vi "DataStream_PC_Main Graph.vi"() -> ()   [LabVIEW 2020]
uses:
  4f3d7b8b-e590-4c89-bcad-6071a54aa44d.vi
  TypeDefs/Cluster_DataStream PC Map Data Set.ctl
panel:
  out "New Update":bool
  out "Cursor Y Diff":dbl
  out "Cursor Time Diff":dbl
  in  "Reset Data":bool
  in  "Pause":bool
  in  "Point Size":i32=2000
  in  "milliseconds to wait":u32=100
  out "Is Connected":bool
  out "Error":errorcluster
  out "error out":errorcluster
  out "XY Graph":cluster{dbl[], dbl[]}[](graph)
  in  "Stop":bool
  in  "Target IP Address":string="172.22.11.2"
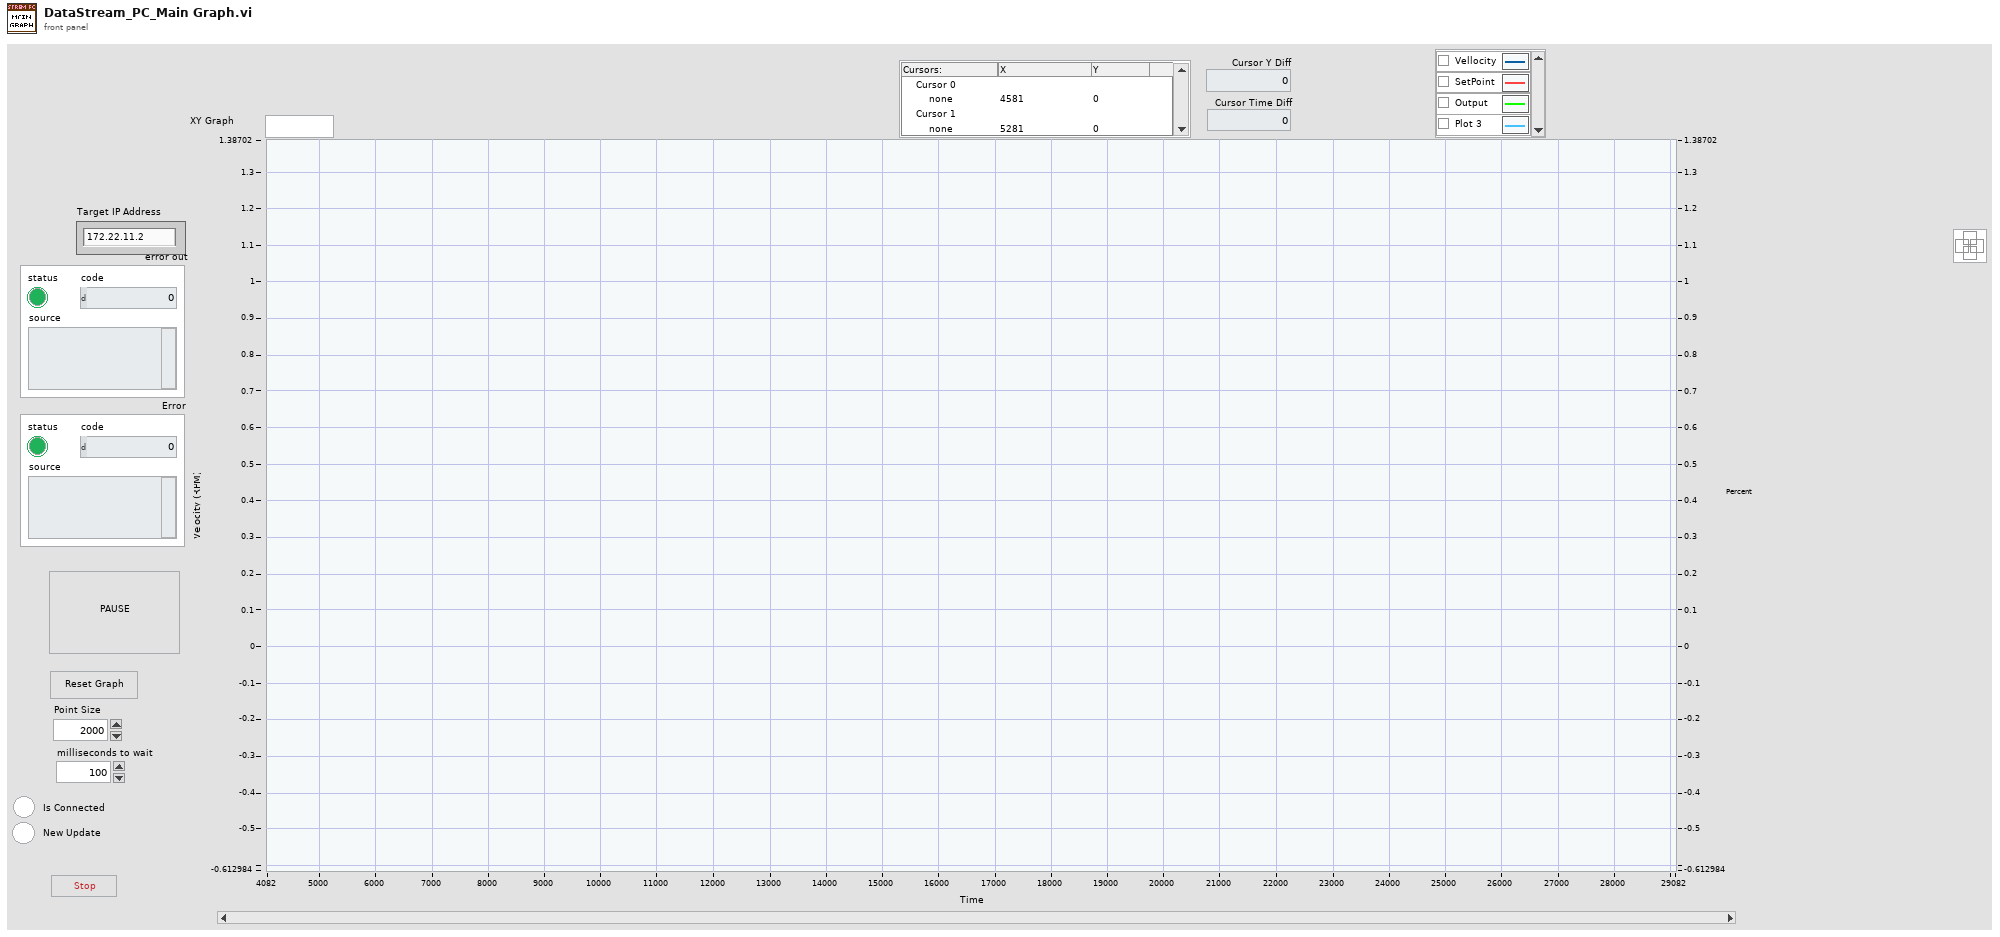
[diagram p1: front panel]
types:
  T1 = typedef "Cluster_DataStream PC Map Data Set.ctl" = cluster{"TimeStamp":dbl[], "Value":dbl[]}
  T2 = typedef "Cluster_DataStream_PC Reader Refs.ctl" = cluster{"Data Reader Ref":refnum<k21>}
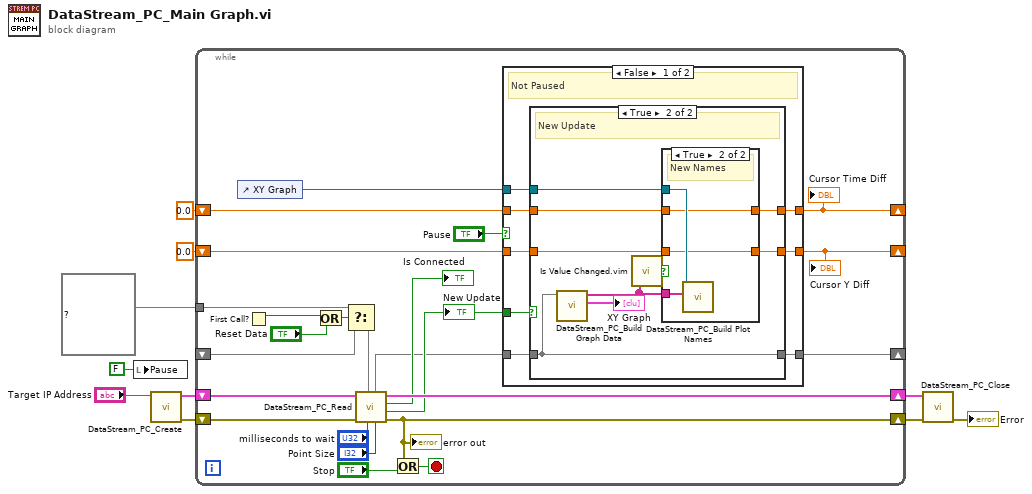
[diagram p0: block diagram]
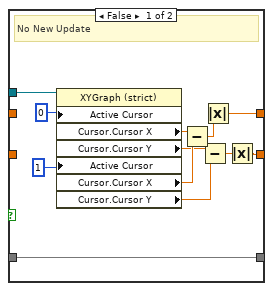
[diagram p2: hidden frame]
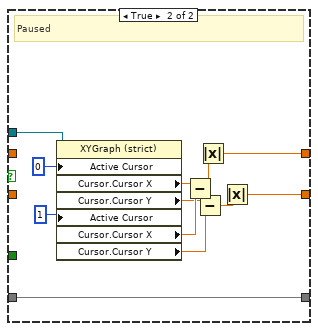
[diagram p4: hidden frame]
diagram:
  n1 = local write "Pause"(FALSE ("Pause")) -> ()
  n2 = call "DataStream_PC_Create.vi"("Target IP Address (10.58.47.2)"="Target IP Address") -> ("Error Out"=w8:errorcluster, "Stream Ref Out"=w9:T2)  [unwired: 9 in]
  n3 = while {
    shift-right: [w31] -> w7
    shift-left: w9 -> [w34]
    shift-right: [w29] -> w6
    shift-left: w8 -> [w33]
    shift-right: [w26] -> _
    shift-left: 0.0 -> [w25]
    shift-right: [w27] -> _
    shift-left: 0.0 -> [w24]
    shift-right: [w19] -> _
    shift-left: _ -> [w17]
    tunnel: map{string, T1} {} ("Map Out") -> [w18]
    stop <- w30 stop-if-true
    n4 = control-ref of="XY Graph"() -> (w23:refnum<vi>)
    n5 = First Call?() -> (First Call?: T/F=w14:bool)
    n6 = Or(x=w14, y="Reset Data") -> (x .or. y?=w15:bool)
    n7 = Select(t=w18, s=w15, f=w17) -> (s? t:f=w16:map{string, T1})
    n8 = call "DataStream_PC_Read.vi"("Point Size"="Point Size", "Milliseconds To Wait"="milliseconds to wait", "Map"=w16, "Error"=w33, "Stream Ref"=w34) -> ("Error Out"=w29:errorcluster, "New Update Out"=w21:bool, "Connected Out"=→"Is Connected":bool, "Stream Ref Out"=w31:T2, "Map Out"=w20:map{string, T1})  [unwired: 2 in]
    "error out" <- w29
    "New Update" <- w21
    n9 = Or(x=w29, y="Stop") -> (x .or. y?=w30:bool)
    n10 = case shown="False" "Pause" {
      tunnel: w21 -> [w42 _]
      tunnel: [w40 w73] -> w27
      tunnel: [w38 w72] -> w26
      tunnel: w25 -> [w39 _]
      tunnel: w24 -> [w41 _]
      tunnel: w23 -> [w37 w71]
      tunnel: w20 -> [w36 w70]
      tunnel: [w35 w70] -> w19
      frame False {
        # "Not Paused"
        n11 = case shown="True" w42 {
          tunnel: w41 -> [_ w56]
          tunnel: [w45 w57] -> w40
          tunnel: w39 -> [_ w59]
          tunnel: [w46 w58] -> w38
          tunnel: w37 -> [w44 w60]
          tunnel: w36 -> [w43 w55]
          tunnel: [w43 w55] -> w35
          frame False {
            # "No New Update"
            n12 = property on="Property Node" class="XYGraph (strict)"(reference=w44, "Active Cursor"=u32 0, "Active Cursor"=u32 1) -> ("Cursor.Cursor X"=w54:dbl, "Cursor.Cursor Y"=w52:dbl, "Cursor.Cursor X"=w53:dbl, "Cursor.Cursor Y"=w51:dbl)  [unwired: 1 in, 2 out]
            n13 = Subtract(x=w54, y=w53) -> (x-y=w50:dbl)
            n14 = Subtract(x=w52, y=w51) -> (x-y=w49:dbl)
            n15 = Absolute Value(x=w50) -> (abs(x)=w46:dbl)
            n16 = Absolute Value(x=w49) -> (abs(x)=w45:dbl)
          }
          frame True {
            # "New Update"
            n17 = call "DataStream_PC_Build Graph Data.vi"("Map"=w55) -> ("Graph Data Out"=→"XY Graph":cluster{"Array":dbl[], "Array":dbl[]}[], "Name Array Out"=w61:string[])  [unwired: 9 in]
            n18 = call "Is Value Changed.vim"("value"=w61) -> ("changed or first call?"=w62:bool)
            n19 = case shown="True" w62 {
              tunnel: w61 -> [_ w69]
              tunnel: w60 -> [_ w68]
              tunnel: w59 -> [w65 w67]
              tunnel: [w65 w67] -> w58
              tunnel: w56 -> [w64 w66]
              tunnel: [w64 w66] -> w57
              frame False {
                # "Same Names"
              }
              frame True {
                # "New Names"
                n20 = call "DataStream_PC_Build Plot Names.vi"("Name Array Out"=w69, "XYGraph in"=w68) -> ()  [unwired: 10 in]
              }
            }
          }
        }
      }
      frame True {
        # "Paused"
        n21 = property on="Property Node" class="XYGraph (strict)"(reference=w71, "Active Cursor"=u32 0, "Active Cursor"=u32 1) -> ("Cursor.Cursor X"=w81:dbl, "Cursor.Cursor Y"=w79:dbl, "Cursor.Cursor X"=w80:dbl, "Cursor.Cursor Y"=w78:dbl)  [unwired: 1 in, 2 out]
        n22 = Subtract(x=w81, y=w80) -> (x-y=w77:dbl)
        n23 = Subtract(x=w79, y=w78) -> (x-y=w76:dbl)
        n24 = Absolute Value(x=w77) -> (abs(x)=w72:dbl)
        n25 = Absolute Value(x=w76) -> (abs(x)=w73:dbl)
      }
    }
    "Cursor Time Diff" <- w26
    "Cursor Y Diff" <- w27
  }
  n26 = call "DataStream_PC_Close.vi"("Error"=w6, "Stream Ref"=w7) -> ("Error Out"=→"Error":errorcluster)  [unwired: 9 in]
